vi "ex10.vi"() -> ()   [LabVIEW 2022 SP3]
panel:
  out "x2":dbl
  out "x1":dbl
  out "Delta":dbl
  in  "c":dbl
  in  "b":dbl
  in  "a":dbl
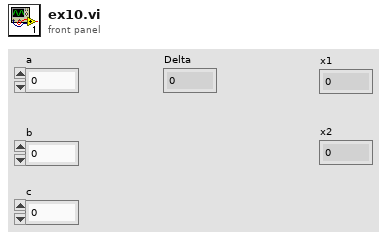
[diagram p1: front panel]
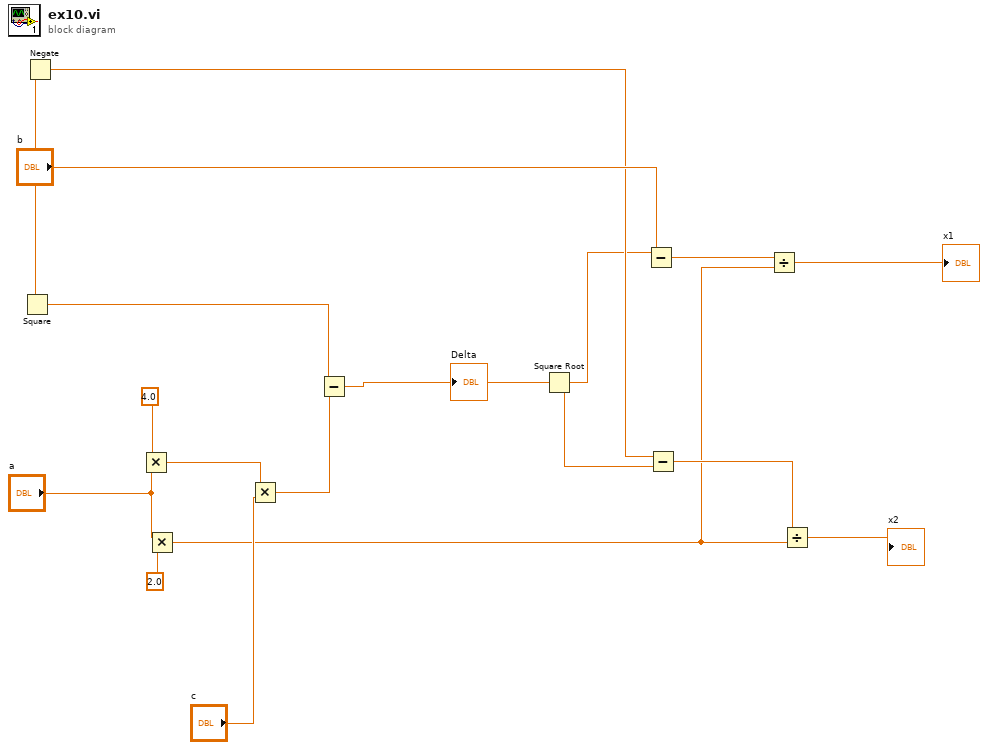
[diagram p0: block diagram]
diagram:
  n1 = Square(x="b") -> (x^2=w12:dbl)
  n2 = Negate(x="b") -> (-x=w5:dbl)
  n3 = Multiply(x=4.0, y="a") -> (x*y=w15:dbl)
  n4 = Multiply(x="a", y=2.0) -> (x*y=w2:dbl)
  n5 = Multiply(x=w15, y="c") -> (x*y=w13:dbl)
  n6 = Subtract(x=w12, y=w13) -> (x-y=w11:dbl)
  "Delta" <- w11
  n7 = Square Root(x=w11) -> (sqrt(x)=w4:dbl)
  n8 = Subtract(x=w4, y="b") -> (x-y=w10:dbl)
  n9 = Subtract(x=w5, y=w4) -> (x-y=w3:dbl)
  n10 = Divide(x=w10, y=w2) -> (x/y=→"x1":dbl)
  n11 = Divide(x=w3, y=w2) -> (x/y=→"x2":dbl)
